vi "LinearFilter_New.vi"(9 "OutputGains":dbl[](array[numeric]) format="%13.5p", 11 "InputGains":dbl[](array[numeric]) format="%13.5p") -> (3 "LINEAR_FILTER":T1 {"Outputs" format="%13.5g"; "Inputs" format="%13.5g"; "OutputGains" format="%13.5g"; "InputGains" format="%13.5g"})   [LabVIEW 2019, in "Trajectory_Library.lvlib"]
doc: "This VI creates a new data structure (cluster) that stores the data for a set of Vis that implement a linear, digital filter. All types of FIR and IIR filters are supported. A set of VIs are provided to create commonly used types of filters.\n \nFilters are of the form: \n y[n] = (b0*x[n] + b1*x[n-1] + ... + bP*x[n-P]) - (a0*y[n-1] + a2*y[n-2] + ... + aQ*y[n-Q])\n \nWhere: \ny[n] is the output at time \"n\" \nx[n] is the input at time \"n\" \ny[n-1] is the output from the LAST time step (\"n-1\") \nx[n-1] is the input from the LAST time step (\"n-1\") \nb0...bP are the \"feedforward\" (FIR) gains \na0...aQ are the \"feedback\" (IIR) gains \n\nIMPORTANT! Note the \"-\" sign in front of the feedback term! This is a common convention in signal processing.\n \nWhat can linear filters do? Basically, they can filter, or diminish, the effects of undesirable input frequencies. High frequencies, or rapid changes, can be indicative of sensor noise or be otherwise undesirable. A \"low pass\" filter smooths out the signal, reducing the impact of these high frequency components. Likewise, a \"high pass\" filter gets rid of slow-moving signal components, letting you detect large changes more easily.\n \nExample FRC applications of filters: \n- Getting rid of noise from an analog sensor input (note: the roboRIO's FPGA can do this faster in hardware)\n- Smoothing out joystick input to prevent the wheels from slipping or the robot from tipping\n- Smoothing motor commands so that unnecessary strain isn't put on electrical or mechanical components\n- If you use clever gains, you can make a PID controller out of this class! (Use the PID set of VI’s instead...)\n \nFor more on filters, we highly recommend the following articles:\n https://en.wikipedia.org/wiki/Linear_filter\n https://en.wikipedia.org/wiki/Iir_filter\n https://en.wikipedia.org/wiki/Fir_filter\n \nNote 1: calculate() should be called by the user on a known, regular period. You can use code in a periodic function.\n \nNote 2: For ALL filters, gains are necessarily a function of frequency. If you make a filter that works well for you at, say, 100Hz, (executing every 10 milliseconds ), you will most definitely need to adjust the gains if you then want to run it at 200Hz, (executing every 5 milliseconds)! Combining this with Note 1, the impetus is on YOU as a developer to make sure calculate() gets called at the desired, constant frequency!\n\nInputs: \n - InputGains - Array of “feedforward” or FIR gain factors (bx)\n\n - OutputGains - Array of “feedback” or IIR gain factors for feedback terms (ax)\n\nOutputs:\n - LINEAR FILTER - cluster containing:\n - InputGains - Array of “feedforward” or FIR gain factors (bx)\n - OutputGains - Array of “feedback” or IIR gain factors for feedback terms (ax)\n - Inputs - Array of the last n saved inputs\n - Outputs - Array of the last n saved outputs\n - InGainCount - Number of input gain terms\n - OutGainCount - number of output gain terms"
uses:
  Trajectory_Library.lvlib
  LINEAR_FILTER.ctl
  <vilib>/Rock Robotics/SystemInterfaces/NetworkCommunication/NetComm_UsageReport_ResourceType.ctl
  Util_LibraryGlobals.vi
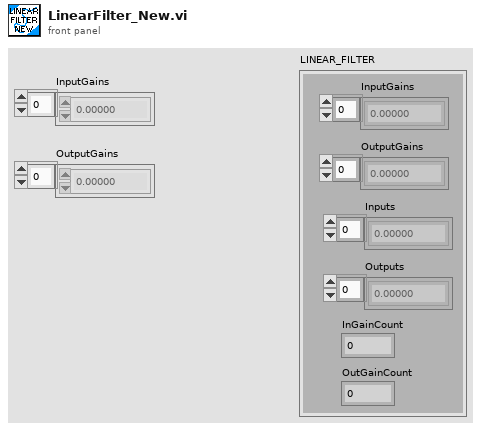
[diagram p1: front panel]
types:
  T1 = typedef "Trajectory_Library.lvlib/LINEAR_FILTER.ctl" = cluster{"InputGains":dbl[], "OutputGains":dbl[], "Inputs":dbl[], "Outputs":dbl[], "InGainCount":i32, "OutGainCount":i32}
  T2 = typedef "NetComm_UsageReport_ResourceType.ctl" = enum8{"Controller", "Module", "Language", "CANPlugin", "Accelerometer", "ADXL345", "AnalogChannel", "AnalogTrigger", "AnalogTriggerOutput", "CANJaguar", "Compressor", "Counter", "Dashboard", "DigitalInput", "DigitalOutput", "DriverStationCIO", "DriverStationEIO", "DriverStationLCD", "Encoder", "GearTooth", "Gyro", "I2C", "Framework", "Jaguar", "Joystick", "Kinect", "KinectStick", "PIDController", "Preferences", "PWM", "Relay", "RobotDrive", "SerialPort", "Servo", "Solenoid", "SPI", "Task", "Ultrasonic", "Victor", "Button", "Command", "AxisCamera", "PCVideoServer", "SmartDashboard", "Talon", "HiTechnicColorSensor", "HiTechnicAccel", "HiTechnicCompass", "SRF08", "AnalogOutput", "Victor SP", "Talon SRX", "CAN Talon SRX", "ADXL362 Accel", "ADXRS450 Gyro", "Rev SPARK", "Mindsensors SD540", "Digital Filter", "ADIS16448", "PDP", "PCM", "PigeonIMU", "Nidec Brushless", "CTRE CANifier", "CTRE TalonFX", "CTRE Future 1", "CTRE Future 2", "CTRE Future 3", "CTRE Future 4", "CTRE Future 5", "CTRE Future 6", "Linear Filter", "Xbox Controller", "USB Camera", "NavX", "Pixy", "Pixy2", "ScanseSweep", "Shuffleboard", "CAN", "Digilent DMC60", "PWM Victor SPX", "Rev SPARK MAX PWM", "Rev SPARK MAX CAN", "ADIS16470", "PIDController2", "ProfiledPIDController", "Kinematics", "Odometry", "Units", "Trapezoid Profile", "DutyCycle", "Addressable LEDs", "Fusion Venom"}
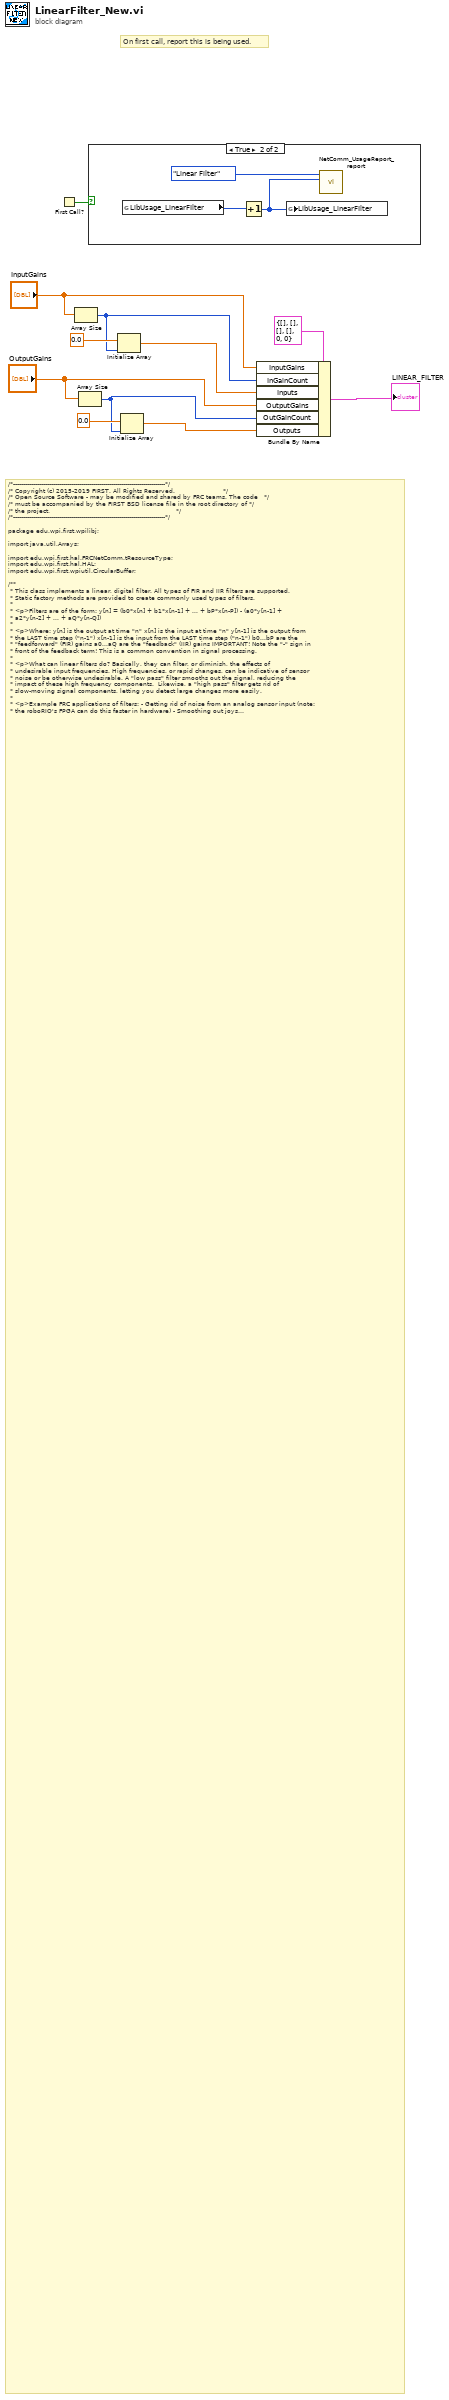
[diagram p0: block diagram]
diagram:
  # "On first call, report this is being used."
  # "/*----------------------------------------------------------------------------*/\n/* Copyright (c) 2015-2019 FIRST. All Rights Reserved.                        */\n/* Open Source Software - may be modified and shared by FRC teams. The code   */\n/* must be accompanied by the FIRST BSD license file in the root directory of */\n/* the project.                                                               */\n/*----------------------------------------------------------------------------*/\n\npackage edu.wpi.first.wpilibj;\n\nimport java.util.Arrays;\n\nimport edu.wpi.first.hal.FRCNetComm.tResourceType;\nimport edu.wpi.first.hal.HAL;\nimport edu.wpi.first.wpiutil.CircularBuffer;\n\n/**\n * This class implements a linear, digital filter. All types of FIR and IIR filters are supported.\n * Static factory methods are provided to create commonly used types of filters.\n *\n * <p>Filters are of the form: y[n] = (b0*x[n] + b1*x[n-1] + ... + bP*x[n-P]) - (a0*y[n-1] +\n * a2*y[n-2] + ... + aQ*y[n-Q])\n *\n * <p>Where: y[n] is the output at time \"n\" x[n] is the input at time \"n\" y[n-1] is the output from\n * the LAST time step (\"n-1\") x[n-1] is the input from the LAST time step (\"n-1\") b0...bP are the\n * \"feedforward\" (FIR) gains a0...aQ are the \"feedback\" (IIR) gains IMPORTANT! Note the \"-\" sign in\n * front of the feedback term! This is a common convention in signal processing.\n *\n * <p>What can linear filters do? Basically, they can filter, or diminish, the effects of\n * undesirable input frequencies. High frequencies, or rapid changes, can be indicative of sensor\n * noise or be otherwise undesirable. A \"low pass\" filter smooths out the signal, reducing the\n * impact of these high frequency components.  Likewise, a \"high pass\" filter gets rid of\n * slow-moving signal components, letting you detect large changes more easily.\n *\n * <p>Example FRC applications of filters: - Getting rid of noise from an analog sensor input (note:\n * the roboRIO's FPGA can do this faster in hardware) - Smoothing out joystick input to prevent the\n * wheels from slipping or the robot from tipping - Smoothing motor commands so that unnecessary\n * strain isn't put on electrical or mechanical components - If you use clever gains, you can make a\n * PID controller out of this class!\n *\n * <p>For more on filters, we highly recommend the following articles:<br>\n * https://en.wikipedia.org/wiki/Linear_filter<br>\n * https://en.wikipedia.org/wiki/Iir_filter<br>\n * https://en.wikipedia.org/wiki/Fir_filter<br>\n *\n * <p>Note 1: calculate() should be called by the user on a known, regular period. You can use a\n * Notifier for this or do it \"inline\" with code in a periodic function.\n *\n * <p>Note 2: For ALL filters, gains are necessarily a function of frequency. If you make a filter\n * that works well for you at, say, 100Hz, you will most definitely need to adjust the gains if you\n * then want to run it at 200Hz! Combining this with Note 1 - the impetus is on YOU as a developer\n * to make sure calculate() gets called at the desired, constant frequency!\n */\npublic class LinearFilter {\n  private final CircularBuffer m_inputs;\n  private final CircularBuffer m_outputs;\n  private final double[] m_inputGains;\n  private final double[] m_outputGains;\n\n  private static int instances;\n\n  /**\n   * Create a linear FIR or IIR filter.\n   *\n   * @param ffGains The \"feed forward\" or FIR gains.\n   * @param fbGains The \"feed back\" or IIR gains.\n   */\n  public LinearFilter(double[] ffGains, double[] fbGains) {\n    m_inputs = new CircularBuffer(ffGains.length);\n    m_outputs = new CircularBuffer(fbGains.length);\n    m_inputGains = Arrays.copyOf(ffGains, ffGains.length);\n    m_outputGains = Arrays.copyOf(fbGains, fbGains.length);\n\n    instances++;\n    HAL.report(tResourceType.kResourceType_LinearFilter, instances);\n  }\n\n  /**\n   * Creates a one-pole IIR low-pass filter of the form: y[n] = (1-gain)*x[n] + gain*y[n-1] where\n   * gain = e^(-dt / T), T is the time constant in seconds.\n   *\n   * <p>This filter is stable for time constants greater than zero.\n   *\n   * @param timeConstant The discrete-time time constant in seconds.\n   * @param period       The period in seconds between samples taken by the user.\n   */\n  public static LinearFilter singlePoleIIR(double timeConstant,\n                                           double period) {\n    double gain = Math.exp(-period / timeConstant);\n    double[] ffGains = {1.0 - gain};\n    double[] fbGains = {-gain};\n\n    return new LinearFilter(ffGains, fbGains);\n  }\n\n  /**\n   * Creates a first-order high-pass filter of the form: y[n] = gain*x[n] + (-gain)*x[n-1] +\n   * gain*y[n-1] where gain = e^(-dt / T), T is the time constant in seconds.\n   *\n   * <p>This filter is stable for time constants greater than zero.\n   *\n   * @param timeConstant The discrete-time time constant in seconds.\n   * @param period       The period in seconds between samples taken by the user.\n   */\n  public static LinearFilter highPass(double timeConstant,\n                                      double period) {\n    double gain = Math.exp(-period / timeConstant);\n    double[] ffGains = {gain, -gain};\n    double[] fbGains = {-gain};\n\n    return new LinearFilter(ffGains, fbGains);\n  }\n\n  /**\n   * Creates a K-tap FIR moving average filter of the form: y[n] = 1/k * (x[k] + x[k-1] + ... +\n   * x[0]).\n   *\n   * <p>This filter is always stable.\n   *\n   * @param taps The number of samples to average over. Higher = smoother but slower.\n   * @throws IllegalArgumentException if number of taps is less than 1.\n   */\n  public static LinearFilter movingAverage(int taps) {\n    if (taps <= 0) {\n      throw new IllegalArgumentException(\"Number of taps was not at least 1\");\n    }\n\n    double[] ffGains = new double[taps];\n    for (int i = 0; i < ffGains.length; i++) {\n      ffGains[i] = 1.0 / taps;\n    }\n\n    double[] fbGains = new double[0];\n\n    return new LinearFilter(ffGains, fbGains);\n  }\n\n  /**\n   * Reset the filter state.\n   */\n  public void reset() {\n    m_inputs.clear();\n    m_outputs.clear();\n  }\n\n  /**\n   * Calculates the next value of the filter.\n   *\n   * @param input Current input value.\n   *\n   * @return The filtered value at this step\n   */\n  public double calculate(double input) {\n    double retVal = 0.0;\n\n    // Rotate the inputs\n    m_inputs.addFirst(input);\n\n    // Calculate the new value\n    for (int i = 0; i < m_inputGains.length; i++) {\n      retVal += m_inputs.get(i) * m_inputGains[i];\n    }\n    for (int i = 0; i < m_outputGains.length; i++) {\n      retVal -= m_outputs.get(i) * m_outputGains[i];\n    }\n\n    // Rotate the outputs\n    m_outputs.addFirst(retVal);\n\n    return retVal;\n  }\n}"
  n1 = First Call?() -> (First Call?: T/F=w1:bool)
  n2 = Array Size(array="InputGains") -> (size(s)=w6:i32)
  n3 = Array Size(array="OutputGains") -> (size(s)=w3:i32)
  n4 = case shown="True" w1 {
    frame False {
    }
    frame True {
      n5 = global read "Util_LibraryGlobals.vi" "LibUsage_LinearFIlter"() -> (w13:i32)
      n6 = Increment(x=w13) -> (x+1=w12:i32)
      n7 = global write "Util_LibraryGlobals.vi" "LibUsage_LinearFIlter"(w12) -> ()
      n8 = call <vilib>:"NetComm_UsageReport_report.vi"("Instance Number"=w12, "Resource Type"=NetComm_UsageReport_ResourceType."Linear Filter") -> ()  [unwired: 10 in]
    }
  }
  n9 = Initialize Array(0.0, w6) -> (w5:dbl[])
  n10 = Initialize Array(0.0, w3) -> (w2:dbl[])
  n11 = Bundle By Name(cluster=T1 {"InputGains"=[], "OutputGains"=[], "Inputs"=[], "Outputs"=[], "InGainCount"=0, "OutGainCount"=0} ("LINEAR_FILTER"), "InputGains"="InputGains", "InGainCount"=w6, "Inputs"=w5, "OutputGains"="OutputGains", "OutGainCount"=w3, "Outputs"=w2) -> (→"LINEAR_FILTER":T1)
